vi "Agilent 681x Standard Triggered Output.vi"() -> ()   [LabVIEW 2019]
doc: "Demonstrates how to use the output triggering system to change output voltage with a trigger."
uses:
  <instrlib>/Agilent 681x Series/Agilent 681x Series.lvlib
panel:
  in  "Pulse Characteristic Value (50)":dbl=50.0 format="%#.4g"
  in  "Pulse Characteristic (0: Duty Cycle)":u16(ring) items=["Duty Cycle", "Pulse Width"]
  in  "Period (0.0333 s)":dbl=0.03333 format="%#.4g"
  in  "Pulse Count (1)":dbl=1.0 format="%#.4g"
  in  "Trigger Delay (0 s)":dbl format="%#.5g"
  in  "Voltage Mode (0: Fix)":u16(ring) items=["Fixed", "Step", "Pulse", "List"]
  in  "Voltage Amplitude (1.0 V)":dbl=1.0 format="%#.4g"
  in  "Triggered Voltage Amplitude (1.0 V)":dbl=1.0 format="%#.4g"
  in  "Serial Configuration":T1={"Baud Rate"=9600, "Parity"=0, "Data Bits"=7} {"Data Bits" items=["7"=7, "8"=8]; "Parity" items=["None", "Odd", "Even", "Mark", "Space"]; "Baud Rate" items=["300"=300, "600"=600, "1200"=1200, "2400"=2400, "4800"=4800, "9600"=9600]}
  in  "VISA resource name":refnum<visa-resource-name>
  # "(c) 2008-2021 National Instruments Corp.  ALL RIGHTS RESERVED."
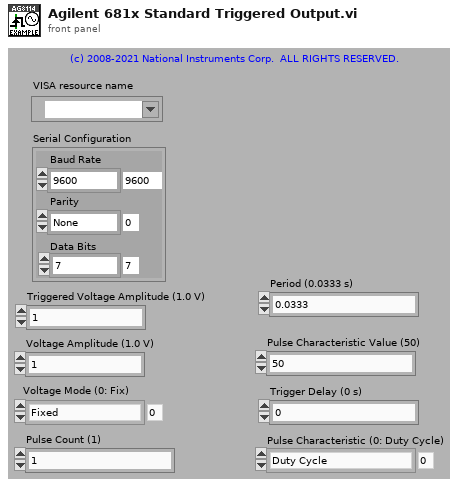
[diagram p1: front panel]
types:
  T1 = cluster{"Baud Rate":u32, "Parity":u16, "Data Bits":u16}
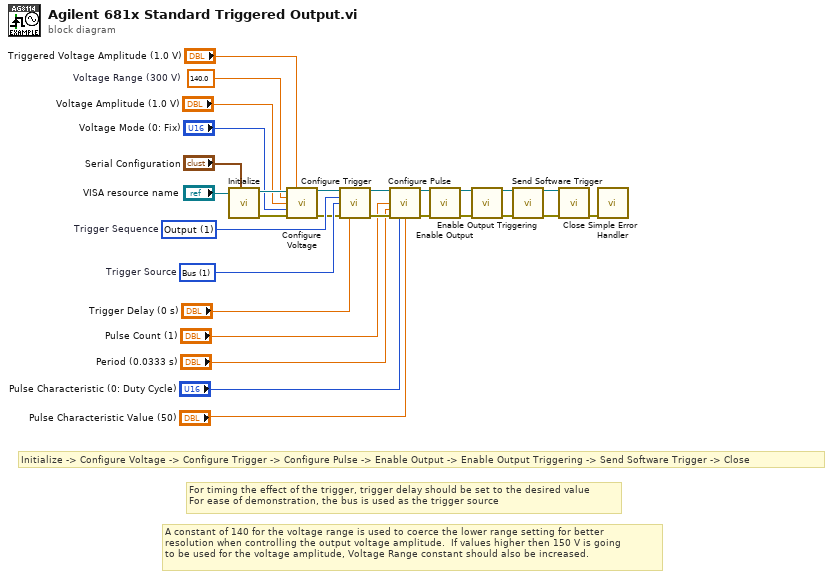
[diagram p0: block diagram]
diagram:
  w20 = 1 items=["Immediate", "Bus", "External", "Phase", "Trigger Out"]  # Trigger Source
  w21 = 1 items=["Output"=1, "Synchronous Source"=2, "Measurement"=3]  # Trigger Sequence
  w24 = 140.0  # Voltage Range (300 V)
  # "For timing the effect of the trigger, trigger delay should be set to the desired value\nFor ease of demonstration, the bus is used as the trigger source"
  # "Initialize -> Configure Voltage -> Configure Trigger -> Configure Pulse -> Enable Output -> Enable Output Triggering -> Send Software Trigger -> Close"
  # "A constant of 140 for the voltage range is used to coerce the lower range setting for better\nresolution when controlling the output voltage amplitude.  If values higher then 150 V is going\nto be used for the voltage amplitude, Voltage Range constant should also be increased."
  n1 = call <instrlib>:"Initialize.vi"("Serial Configuration"="Serial Configuration", "VISA resource name"="VISA resource name") -> ("error out"=w25:errorcluster, "VISA resource name out"=w26:refnum<visa-resource-name>)  [unwired: 8 in]
  n2 = call <instrlib>:"Configure Voltage.vi"("VISA resource name"=w26, "Triggered Voltage Amplitude (1.0 V)"="Triggered Voltage Amplitude (1.0 V)", "Voltage Range (300 V)"=w24, "Voltage Amplitude (1.0 V)"="Voltage Amplitude (1.0 V)", "Voltage Mode (0: Fix)"="Voltage Mode (0: Fix)", "error in (no error)"=w25) -> ("VISA resource name out"=w12:refnum<visa-resource-name>, "error out"=w13:errorcluster)  [unwired: 8 in]
  n3 = call <instrlib>:"Configure Trigger.vi"("VISA resource name"=w12, "Trigger Sequence (1: Output 1)"=w21, "Trigger Source (0: Immediate)"=w20, "error in (no error)"=w13, "Trigger Delay (0 s)"="Trigger Delay (0 s)") -> ("VISA resource name out"=w18:refnum<visa-resource-name>, "error out"=w19:errorcluster)  [unwired: 9 in]
  n4 = call <instrlib>:"Configure Pulse.vi"("VISA resource name"=w18, "Pulse Count (1)"="Pulse Count (1)", "Period (0.0333 s)"="Period (0.0333 s)", "error in (no error)"=w19, "Pulse Characteristic (0: Duty Cycle)"="Pulse Characteristic (0: Duty Cycle)", "Pulse Characteristic Value (50)"="Pulse Characteristic Value (50)") -> ("VISA resource name out"=w16:refnum<visa-resource-name>, "error out"=w17:errorcluster)  [unwired: 8 in]
  n5 = call <instrlib>:"Enable Output.vi"("VISA resource name"=w16, "error in (no error)"=w17) -> ("VISA resource name out"=w23:refnum<visa-resource-name>, "error out"=w22:errorcluster)  [unwired: 12 in]
  n6 = call <instrlib>:"Enable Output Triggering.vi"("VISA resource name"=w23, "error in (no error)"=w22) -> ("VISA resource name out"=w15:refnum<visa-resource-name>, "error out"=w14:errorcluster)  [unwired: 12 in]
  n7 = call <instrlib>:"Send Software Trigger.vi"("VISA resource name"=w15, "error in (no error)"=w14) -> ("VISA resource name out"=w10:refnum<visa-resource-name>, "error out"=w11:errorcluster)  [unwired: 12 in]
  n8 = call <instrlib>:"Close.vi"("error in (no error)"=w11, "VISA resource name"=w10) -> ("error out"=w9:errorcluster)  [unwired: 9 in]
  n9 = call <vilib>:"Simple Error Handler.vi"("error in (no error)"=w9) -> ()  [unwired: 4 in, 5 out]
